vi "Sine Function.vi"(1 "Input":dbl) -> (0 "Output":dbl)   [LabVIEW 2015]
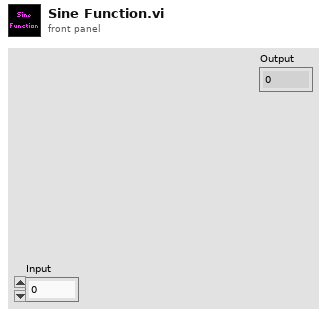
[diagram p1: front panel]
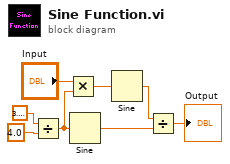
[diagram p0: block diagram]
diagram:
  n1 = Divide(x=3.141592653589793, y=4.0) -> (x/y=w1:dbl)
  n2 = Multiply(x="Input", y=w1) -> (x*y=w2:dbl)
  n3 = Sine(x=w1) -> (sin(x)=w5:dbl)
  n4 = Sine(x=w2) -> (sin(x)=w4:dbl)
  n5 = Divide(x=w4, y=w5) -> (x/y=→"Output":dbl)
